vi "Add VIs and their Protperties to Tree.vi"(5 "Globals?":bool=TRUE, 6 "File Extension Filters":string[](array[string]), 7 "Exclude vi.lib?":bool=TRUE, 8 "error in":errorcluster, 9 "Search Clones Up To":i32=100, 10 "AppInst":refnum<vi>, 11 "Data Tree":refnum<vi>) -> (0 "error out":errorcluster)   [LabVIEW 2013]
doc: "For a given application instance, this VI generates a tree control listing all VIs currently in memory, including all statically-referenced reentrant clones. User supplied filters are then applied. Currently active instances of any asynchronously launched reentrant VIs, which were tagged for inclusion, are also added to the tree. This tagging is accomplished by dropping the \"Clone VIs FG\" DropIn VI onto the block diagram of any reentrant VI which you wish to monitor. These tagged items will not be filtered."
uses:
  Clone VIs FG Enum.ctl
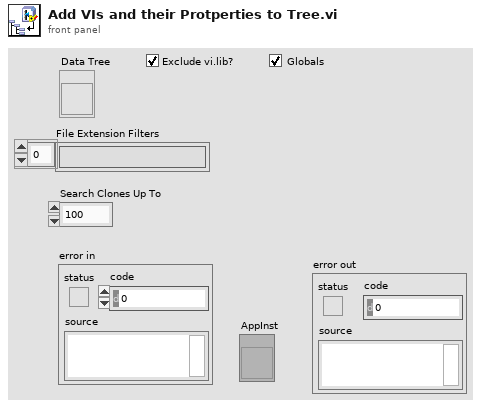
[diagram p1: front panel]
types:
  T1 = typedef "Clone VIs FG Enum.ctl" = enum16{"Get", "Get Active VIs", "Add Calling VI"}
  T2 = enum32{"invalid VI type", "Standard VI", "Control VI", "Global VI", "Polymorphic VI", "Configuration VI", "SubSystem", "Facade VI", "Method VI", "Statechart Diagram VI"}
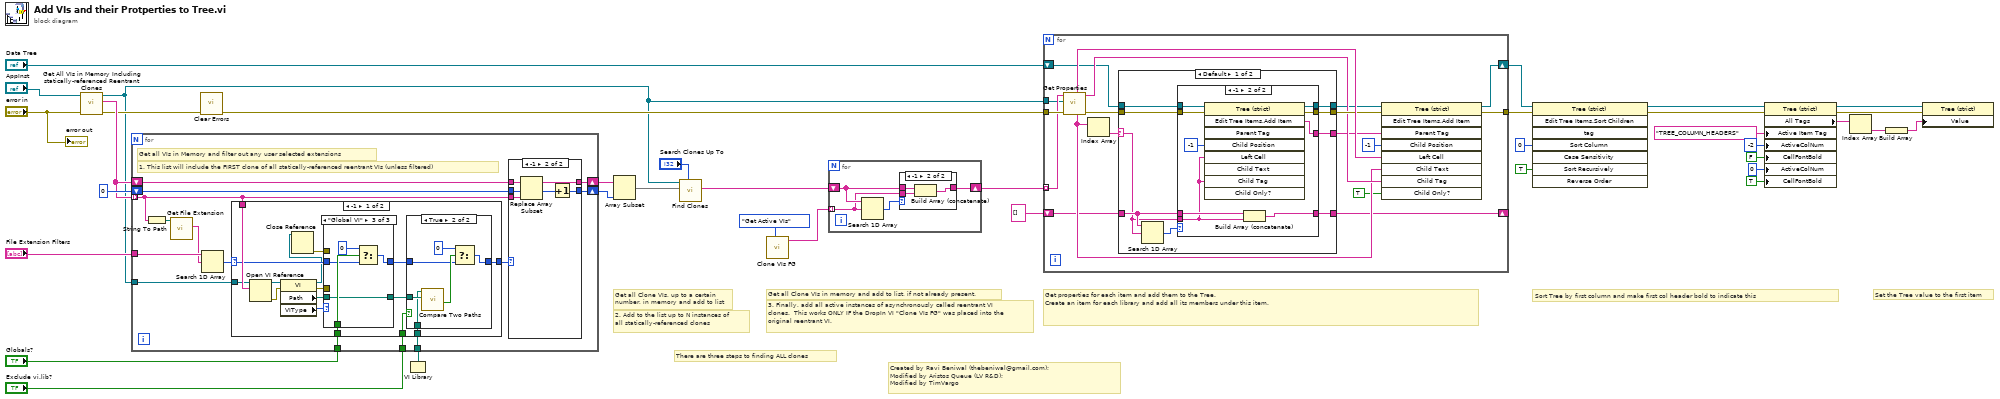
[diagram p0: block diagram]
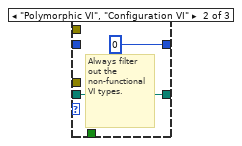
[diagram p5: hidden frame]
diagram:
  # "There are three steps to finding ALL clones"
  # "3. Finally, add all active instances of asynchronously called reentrant VI clones.  This works ONLY IF the DropIn VI \"Clone VIs FG\" was placed into the original reentrant VI."
  # "2. Add to the list up to N instances of all statically-referenced clones"
  # "Get all Clone VIs in memory and add to list, if not already present."
  # "Get all Clone VIs, up to a certain \nnumber, in memory and add to list"
  # "Sort Tree by first column and make first col header bold to indicate this"
  # "Created by Ravi Beniwal (thebeniwal@gmail.com);\nModified by Aristos Queue (LV R&D);\nModified by TimVargo"
  # "Set the Tree value to the first item"
  # "Get properties for each item and add them to the Tree.\nCreate an item for each library and add all its members under this item."
  n1 = call "Get All VIs in Memory Including statically-referenced Reentrant Clones.vi"("error in (no error)"="error in", "App Refnum"="AppInst") -> ("error out"=w10:errorcluster, "All VIs in Memory Including Reentrant Clones"=w12:string[], "App Refnum Out"=w3:refnum<vi>)  [unwired: 7 in]
  n2 = call <vilib>:"Clear Errors.vi"("error in (no error)"=w10) -> ("error out"=w4:errorcluster)  [unwired: 6 in]
  n3 = VI Library() -> (path=w15:path)
  n4 = for {
    tunnel: w12 -> [w42] mode=indexing
    tunnel: "File Extension Filters" -> [w50]
    shift-right: [w47] -> w34
    shift-left: w12 -> [w48]
    shift-right: [w45] -> w33
    shift-left: 0 -> [w46]
    tunnel: "Globals?" -> [w41]
    tunnel: "Exclude vi.lib?" -> [w40]
    tunnel: w15 -> [w39]
    tunnel: w3 -> [w38]
    # "1. This list will include the FIRST clone of all statically-referenced reentrant VIs (unless filtered)"
    # "Get all VIs in Memory and filter out any user selected extensions"
    n5 = String To Path(string=w42) -> (path=w51:path)
    n6 = call <vilib>:"Get File Extension.vi"("file"=w51) -> ("lowercase file extension"=w49:string)  [unwired: 7 in, 3 out]
    n7 = Search 1D Array(1D array=w50, element=w49) -> (index of element=w44:i32)  [unwired: 1 in]
    n8 = case shown="-1" w44 {
      selector: w44 -> [w64 w84]
      tunnel: [w57 w84] -> w43
      tunnel: w42 -> [w67 _]
      tunnel: w41 -> [w62 _]
      tunnel: w40 -> [w61 _]
      tunnel: w39 -> [w59 _]
      tunnel: w38 -> [w52 _]
      frame -1 {
        n9 = Open VI Reference(application reference (local)=w52, vi path=w67) -> (vi reference=w66:refnum<vi>, error out=w55:errorcluster)  [unwired: 4 in]
        n10 = property class="VI"(reference=w66, error in=w55) -> (reference out=w56:refnum<vi>, error out=w54:errorcluster, "Path"=w63:path, "VIType"=w65:T2)
        n11 = Close Reference(reference=w56) -> (error out=w53:errorcluster)  [unwired: 1 in]
        n12 = case shown="\"Global VI\"" w65 {
          tunnel: w64 -> [w76 _ w82]
          tunnel: [w76 0 ("index of element") w81] -> w58
          tunnel: w63 -> [w75 w77 w79]
          tunnel: w62 -> [_ _ w83]
          tunnel: [w75 w77 w79] -> w60
          tunnel: w54 -> [_ _ _]
          tunnel: w53 -> [_ _ _]
          frame Default {
          }
          frame "Polymorphic VI", "Configuration VI" {
            # "Always filter out the non-functional VI types."
          }
          frame "Global VI" {
            n13 = Select(t=0, s=w83, f=w82) -> (s? t:f=w81:i32)
          }
        }
        n14 = case shown="True" w61 {
          tunnel: w60 -> [_ w74]
          tunnel: w59 -> [_ w73]
          tunnel: w58 -> [w68 w71]
          tunnel: [w68 w69] -> w57
          frame False {
          }
          frame True {
            n15 = call <vilib>:"Compare Two Paths.vi"("Path 2"=w74, "Path 1"=w73) -> ("Path 2 Relative to Path 1?"=w72:bool)  [unwired: 6 in, 3 out]
            n16 = Select(t=0, s=w72, f=w71) -> (s? t:f=w69:i32)
          }
        }
      }
      frame Default {
      }
    }
    n17 = case shown="-1" w43 {
      tunnel: w48 -> [w86 w91]
      tunnel: [w86 w90] -> w47
      tunnel: w42 -> [_ w89]
      tunnel: w46 -> [w85 w88]
      tunnel: [w85 w87] -> w45
      frame 0, Default {
      }
      frame -1 {
        n18 = Replace Array Subset(array=w91, new element=w89, index=w88) -> (w90:string[])
        n19 = Increment(x=w88) -> (x+1=w87:i32)
      }
    }
  }
  n20 = Array Subset(array=w34, length=w33) -> (w14:string[])  [unwired: 1 in]
  n21 = call "Find Clones.vi"("Search Clones Up To"="Search Clones Up To", "VIs in"=w14, "Application in"=w3) -> ("VIs (including clones) out"=w6:string[])  [unwired: 8 in]
  n22 = call "Clone VIs FG.vi"("Action"=Clone_VIs_FG_Enum."Get Active VIs") -> ("VIs"=w7:string[])  [unwired: 9 in, 1 out]
  n23 = for {
    shift-right: [w94] -> w5
    shift-left: w6 -> [w95]
    tunnel: w7 -> [w93] mode=indexing
    n24 = Search 1D Array(1D array=w95, element=w93) -> (index of element=w92:i32)  [unwired: 1 in]
    n25 = case shown="-1" w92 {
      tunnel: w95 -> [w96 w99]
      tunnel: [w96 w98] -> w94
      tunnel: w93 -> [_ w97]
      frame 0, Default {
      }
      frame -1 {
        n26 = Build Array (concatenate)(w99, w97) -> (w98:string[])
      }
    }
  }
  n27 = for {
    tunnel: w5 -> [w113] mode=indexing
    tunnel: w4 -> [w116]
    tunnel: [w115] -> w30
    shift-right: [w114] -> w27
    shift-left: "Data Tree" -> [w102]
    tunnel: w3 -> [w111]
    shift-right: [w103] -> _
    shift-left: string[] [] -> [w104]
    n28 = call "Get Properties.vi"("error in"=w116, "AppInst"=w111, "VI Name"=w113) -> ("error out"=w109:errorcluster, "Full Name Out"=w108:string, "VI Properties (All)"=w107:string[], "File Name Out"=w112:string)  [unwired: 2 in, 3 out]
    n29 = Index Array(array=w107) -> (element=w106:string)  [unwired: 1 in]
    n30 = case shown="Default" w106 {
      selector: w106 -> [w118 w143]
      tunnel: [w126 w142] -> w110
      tunnel: w109 -> [w125 w142]
      tunnel: [w119 w143] -> w105
      tunnel: w104 -> [w123 w140]
      tunnel: [w124 w140] -> w103
      tunnel: w102 -> [w122 w141]
      tunnel: [w121 w141] -> w101
      frame Default {
        n31 = Search 1D Array(1D array=w123, element=w118) -> (index of element=w120:i32)  [unwired: 1 in]
        n32 = case shown="-1" w120 {
          tunnel: [w129 w138] -> w126
          tunnel: w125 -> [w129 w137]
          tunnel: [w128 w136] -> w124
          tunnel: w123 -> [w128 w135]
          tunnel: w118 -> [w127 w131]
          tunnel: w122 -> [w130 w134]
          tunnel: [w130 w133] -> w121
          tunnel: [w127 w132] -> w119
          frame 0, Default {
          }
          frame -1 {
            n33 = invoke on="Invoke Node" class="Tree (strict)" method="Edit Tree Items.Add Item"(reference=w134, error in=w137, "Child Position"=-1, "Left Cell"=w131, "Child Tag"=w131) -> (reference out=w133:refnum<vi>, error out=w138:errorcluster, "Edit Tree Items:Add Item"=w132:string)  [unwired: 4 in, 6 out]
            n34 = Build Array (concatenate)(w135, w131) -> (w136:string[])
          }
        }
      }
      frame "" {
      }
    }
    n35 = invoke on="Invoke Node" class="Tree (strict)" method="Edit Tree Items.Add Item"(reference=w101, error in=w110, "Parent Tag"=w105, "Child Position"=-1, "Left Cell"=w112, "Child Text"=w107, "Child Tag"=w108, "Child Only?"=TRUE) -> (reference out=w114:refnum<vi>, error out=w115:errorcluster)  [unwired: 1 in, 7 out]
  }
  n36 = invoke on="Invoke Node" class="Tree (strict)" method="Edit Tree Items.Sort Children"(reference=w27, error in=w30, "Sort Column"=0, "Sort Recursively"=TRUE ("Sort Recursively?")) -> (reference out=w28:refnum<vi>, error out=w29:errorcluster)  [unwired: 4 in, 6 out]
  n37 = property class="Tree (strict)"(reference=w28, error in=w29, "Active Item Tag"="TREE_COLUMN_HEADERS" ("Active Item:Tag"), "ActiveColNum"=-2 ("Active Cell:Active Column Number"), "CellFontBold"=FALSE ("Active Cell:Cell Font:Bold"), "ActiveColNum"=0 ("Active Cell:Active Column Number"), "CellFontBold"=TRUE ("Active Cell:Cell Font:Bold")) -> (reference out=w24:refnum<vi>, error out=w25:errorcluster, "All Tags"=w26:string[])
  n38 = Index Array(array=w26) -> (element=w23:string)  [unwired: 1 in]
  n39 = Build Array(w23) -> (w32:string[])
  n40 = property class="Tree (strict)"(reference=w24, error in=w25, "Value"=w32) -> ()  [unwired: 2 out]
  "error out" <- "error in"
